vi "GraphLegendGen.vi"(4 "Plot colors":u32[](array[colorbox])=[16777215, 16711680, 65280, 16776960, 65535, 16711935, 255, 16744448, 8388863, 11645283, 46096, 12632256, 34502, 16711808, 9947136, 11826176, 11796589, 7439103, 15728520, 16764921, 61349, 16764296, 12058457, 10539775, 13872565, 16746727, 41215, 8978944, 16757081, 16766208, 10777087, 10066329, 15000804, 13128704, 16760248, 16742466, 13827929, 46140, 10527356, 16777215, 16711680, 65280, 16776960, 65535, 16711935, 255, 16744448, 8388863, 11645283, 46096, 12632256, 34502, 16711808, 9947136, 11826176, 11796589, 7439103, 15728520, 16764921, 61349, 16764296, 12058457, 10539775, 13872565, 16746727, 41215, 8978944, 16757081, 16766208, 10777087, 10066329, 15000804, 13128704, 16760248, 16742466, 13827929, 46140, 10527356, 16777215, 16711680, 65280, 16776960, 65535, 16711935, 255, 16744448, 8388863, 11645283, 46096, 12632256, 34502, 16711808, 9947136, 11826176, 11796589, 7439103, 15728520, 16764921, 61349, 16764296, 12058457, 10539775, 13872565, 16746727, 41215, 8978944, 16757081, 16766208, 10777087, 10066329, 15000804, 13128704, 16760248, 16742466, 13827929, 46140, 10527356, 16777215, 16711680, 65280, 16776960, 65535, 16711935, 255, 16744448, 8388863, 11645283, 46096, 12632256, 34502, 16711808, 9947136, 11826176, 11796589, 7439103, 15728520, 16764921, 61349, 16764296, 12058457, 10539775, 13872565, 16746727, 41215, 8978944, 16757081, 16766208, 10777087, 10066329, 15000804, 13128704, 16760248, 16742466, 13827929, 46140, 10527356], 5 "LastCrvInd":i32=-1, 6 "error in (no error)":errorcluster, 7 "Scan list":string[](array[string]), 8 "Échelle X":string, 9 "XY Graph Ref":refnum<vi>) -> (0 "error out":errorcluster, 1 "Plot colors Out":u32[](array[colorbox])=[16777215, 16711680, 65280, 16776960, 65535, 16711935, 255, 16744448, 8388863, 11645283, 46096, 12632256, 34502, 16711808, 9947136, 11826176, 11796589, 7439103, 15728520, 16764921, 61349, 16764296, 12058457, 10539775, 13872565, 16746727, 41215, 8978944, 16757081, 16766208, 10777087, 10066329, 15000804, 13128704, 16760248, 16742466, 13827929, 46140, 10527356])   [LabVIEW 2010]
doc: "Ce VI formatte la légende du graphique en fonction des paramètres de balayage choisis."
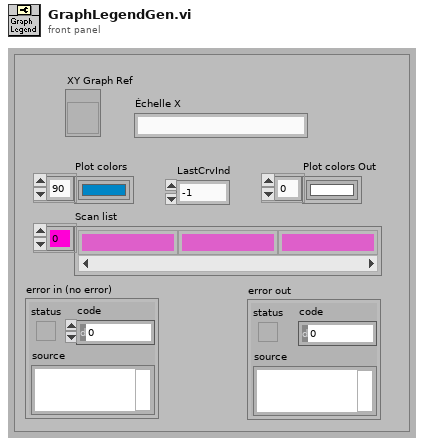
[diagram p1: front panel]
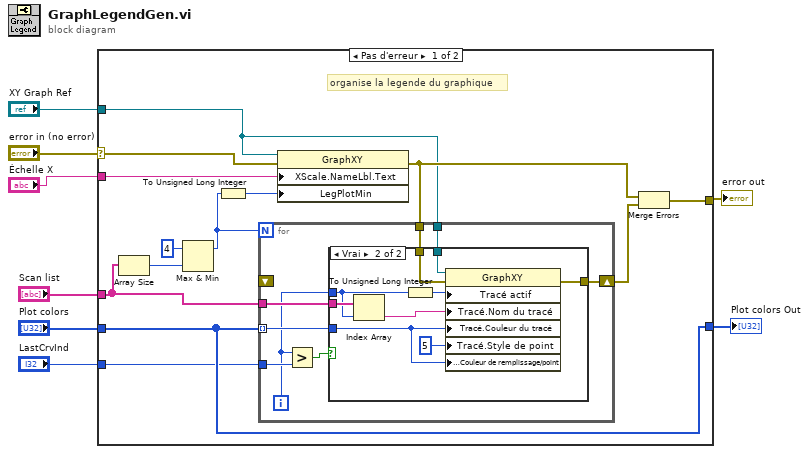
[diagram p0: block diagram]
diagram:
  n1 = case shown="Pas d'erreur" "error in (no error)" {
    selector: "error in (no error)" -> [w10 w41]
    tunnel: "XY Graph Ref" -> [w12 _]
    tunnel: "Scan list" -> [w19 _]
    tunnel: [w20 w41] -> w7
    tunnel: "Plot colors" -> [w13 w40]
    tunnel: [w13 w40] -> w3
    tunnel: "LastCrvInd" -> [w11 _]
    tunnel: "Échelle X" -> [w9 _]
    frame No Error {
      # "organise la legende du graphique"
      n2 = Array Size(array=w19) -> (size(s)=w18:i32)
      n3 = Max & Min(x=4, y=w18) -> (max(x,y)=w15:i32)  [unwired: 1 out]
      n4 = To Unsigned Long Integer(number=w15) -> (unsigned 32bit integer=w14:u32)
      n5 = property class="GraphXY"(reference=w12, error in=w10, "XScale.NameLbl.Text"=w9, "LegPlotMin"=w14) -> (error out=w16:errorcluster)  [unwired: 1 out]
      n6 = for {
        N: w15 -> [_]
        tunnel: w19 -> [w25]
        tunnel: w12 -> [w29]
        tunnel: w13 -> [w26] mode=indexing
        tunnel: w16 -> [w28]
        shift-right: [w27] -> w21
        shift-left: _ -> [_]
        tunnel: w11 -> [w24]
        i -> [w23]
        n7 = Greater?(x=w23, y=w24) -> (0:w22:bool)
        n8 = case shown="Vrai" w22 {
          tunnel: w29 -> [_ w39]
          tunnel: w28 -> [w30 w37]
          tunnel: [w30 w36] -> w27
          tunnel: w26 -> [_ w34]
          tunnel: w23 -> [_ w31]
          tunnel: w25 -> [_ w33]
          frame False {
          }
          frame True {
            n9 = Index Array(array=w33, index=w31) -> (element=w32:string)
            n10 = To Unsigned Long Integer(number=w31) -> (unsigned 32bit integer=w35:u32)
            n11 = property class="GraphXY"(reference=w39, error in=w37, "Tracé actif"=w35, "Tracé.Nom du tracé"=w32, "Tracé.Couleur du tracé"=w34, "Tracé.Style de point"=u8 5 ("Plot.Point Style"), "Tracé.Couleur de remplissage/point"=w34) -> (error out=w36:errorcluster)  [unwired: 1 out]
          }
        }
      }
      n12 = Merge Errors(w16, w21) -> (w20:errorcluster)
    }
    frame Error {
    }
  }
  "error out" <- w7
  "Plot colors Out" <- w3
